vi "BotSpeak_FILE SAVE.vi"(2 "file name":string="test.htm", 3 "HTML text":string="<!DOCTYPE html>\n<html>\n<body>\n\n<h1>My First Heading</h1>\n\n<p>My first paragraph.</p>\n\n</body>\n</html>\n", 4 "Bot Settings":T1) -> (0 "response":string="169.254.32.85", 1 "Bot Settings 2":T1)   [LabVIEW 2014]
doc: "Saves the desired \"HTML text\" to the RIO as the specified \"file name\"."
uses:
  <userlib>/botspeak/VIs/Direct/BotSpeak_Control.ctl
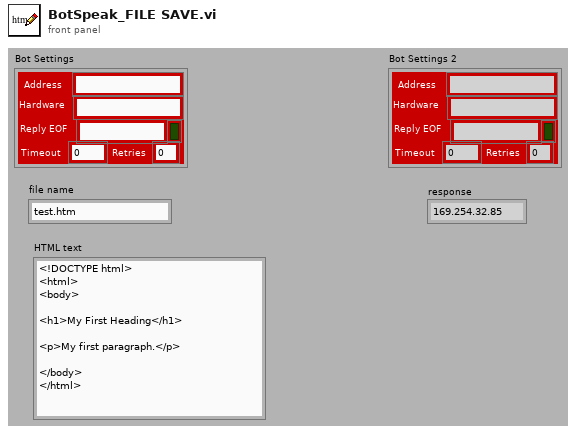
[diagram p1: front panel]
types:
  T1 = typedef "BotSpeak_Control.ctl" = cluster{"Address":string, "Reply EOF":string, "Hardware":string, "Retries":i8, "Timeout":i32, "Open?":bool}
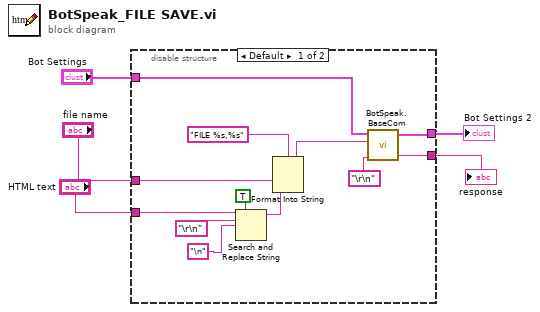
[diagram p0: block diagram]
diagram:
  n1 = disable-structure shown="Default" {
    disable-tunnel: "file name" -> [w16 _]
    disable-tunnel: "HTML text" -> [w14 _]
    disable-tunnel: "Bot Settings" -> [w9 _]
    disable-tunnel: [w8 _] -> w2
    disable-tunnel: [w6 _] -> w1
    frame condition #0 (active) {
      n2 = Search and Replace String(replace all?=TRUE ("replace all? (F)"), input string=w14, search string="\r\n", replace string="\n" ("search string")) -> (result string=w15:string)  [unwired: 4 in, 3 out]
      n3 = Format Into String(format string="FILE %s,%s" ("command"), w16, w15) -> (resulting string=w7:string)  [unwired: 2 in, 1 out]
      n4 = call <userlib>:"BotSpeak.BaseCom.vi"("Termination"="\r\n", "command"=w7, "Bot Settings in"=w9) -> ("response"=w6:string, "Bot Settings out"=w8:T1)  [unwired: 2 in]
    }
    frame condition #1 {
    }
  }
  "Bot Settings 2" <- w2
  "response" <- w1
